vi "Lire Parameters.vi"(11 "Stock en entrée":refnum<class "Stock.lvclass">) -> (2 "Parameters":T1={"Label"="", "Symbol"="SU", "Dividend"=0.0, "Currency"=enum."Euro", "ISIN"="", "Symbol_Suffix"=".PA", "Last Price"=0.0, "Dividend-Date"="", "Change (%)"=0.0, "Objective"=0.0, "Stop"=0.0}, 3 "Stock en sortie":refnum<class "Stock.lvclass">)   [LabVIEW 2012, in "Stock.lvclass"]
uses:
  Stock.lvclass
  Stock Parameters.ctl
  controls/Currencies.ctl
  Stock.lvclass/Stock.ctl
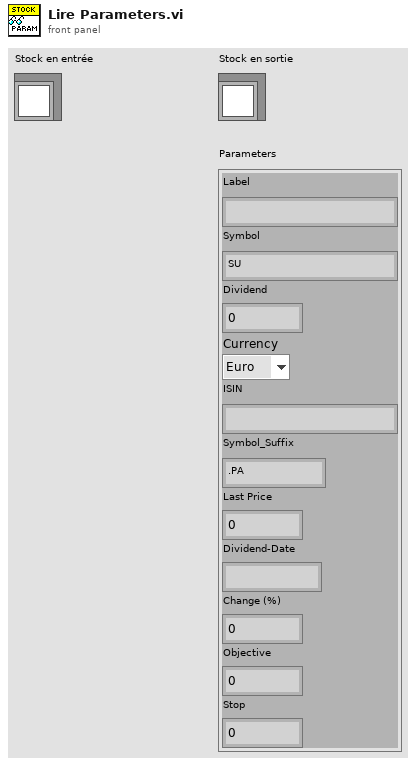
[diagram p1: front panel]
types:
  T1 = typedef "Stock.lvclass/Stock Parameters.ctl" = cluster{"Label":string, "Symbol":string, "Dividend":dbl, "Currency":T2, "ISIN":string, "Symbol_Suffix":string, "Last Price":dbl, "Dividend-Date":string, "Change (%)":dbl, "Objective":dbl, "Stop":dbl}
  T2 = typedef "Currencies.ctl" = enum16{"Euro", "Dollar", "Yen", "RIM", "CHF"}
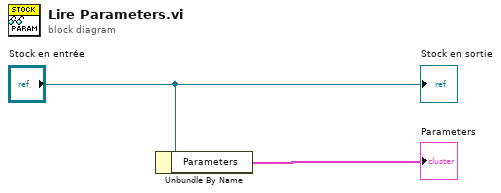
[diagram p0: block diagram]
diagram:
  n1 = Unbundle By Name("Stock en entrée") -> ("Parameters"=→"Parameters":T1)
  "Stock en sortie" <- "Stock en entrée"
